vi "sub_apt_getposition.vi"(8 "错误输入（无错误）":errorcluster, 11 "引用":refnum<k7>) -> (0 "错误输出":errorcluster, 2 "GetPosition_Position":sgl, 3 "引用输出":refnum<k7>)   [LabVIEW 2015]
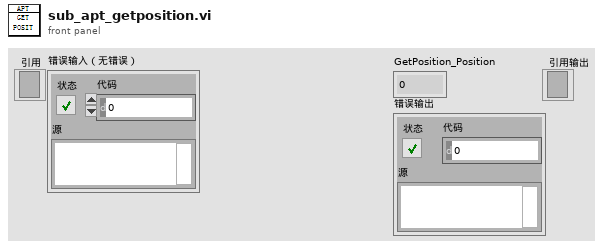
[diagram p1: front panel]
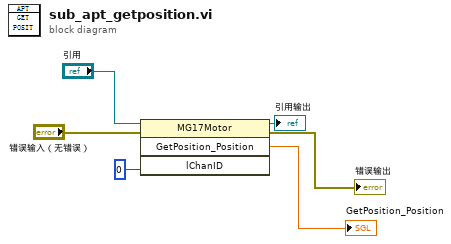
[diagram p0: block diagram]
diagram:
  n1 = invoke class="MG17Motor" method="GetPosition_Position"(reference="引用", error in="错误输入（无错误）", "lChanID"=0) -> (reference out=→"引用输出":refnum<k7>, error out=→"错误输出":errorcluster, "GetPosition_Position"=→"GetPosition_Position":sgl)  [unwired: 1 in, 1 out]
